vi "Write LinearConfig.vi"(8 "error in (no error)":errorcluster, 10 "LinearConfig":T1={"decoding type"=10092, "units"=10219, "distance per pulse"=0.001, "initial position"=0.0, "z index enable"=FALSE, "z index value"=0.0, "z index phase"=10040} {"units" items=["Meters"=10219, "Inches"=10379, "Ticks"=10304, "From Custom Scale"=10065]; "decoding type" items=["X1"=10090, "X2"=10091, "X4"=10092, "Two Pulse Counting"=10313]; "z index phase" items=["A High B High"=10040, "A High B Low"=10041, "A Low B High"=10042, "A Low B Low"=10043]}, 11 "Linear_Task in":refnum<class "Linear_Task.lvclass">) -> (0 "error out":errorcluster, 3 "Linear_Task out":refnum<class "Linear_Task.lvclass">)   [LabVIEW 2025, in "Linear_Task.lvlib" / "Linear_Task.lvclass"]
uses:
  Linear_Task.lvclass
  Linear_Task.lvclass/Linear_Task.ctl
  DAQ_Module/DAQ_Module/DAQ_Module/DAQ_Linear_Task_Config.ctl
  DAQ_Module/DAQ_Module/DAQ_Module/DAQ_Module.lvclass
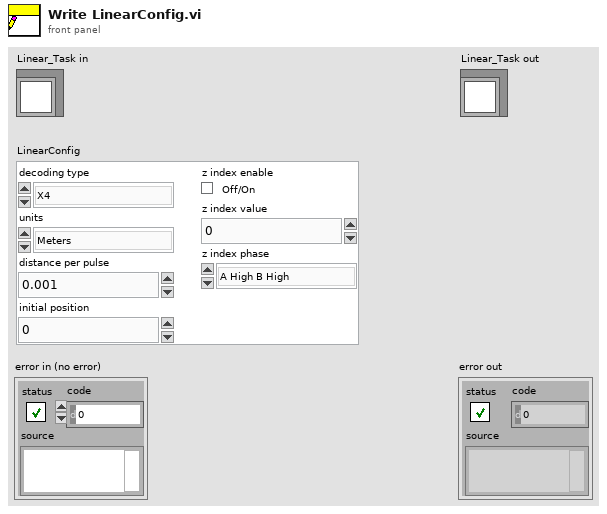
[diagram p1: front panel]
types:
  T1 = typedef "DAQ_Module.lvlib/DAQ_Module.lvclass/DAQ_Linear_Task_Config.ctl" = cluster{"decoding type":i32, "units":i32, "distance per pulse":dbl, "initial position":dbl, "z index enable":bool, "z index value":dbl, "z index phase":i32}
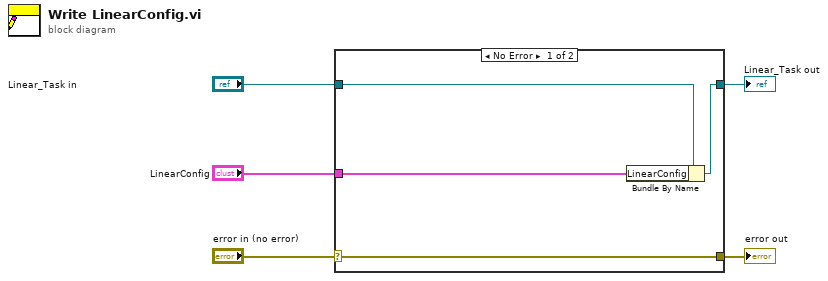
[diagram p0: block diagram]
diagram:
  n1 = case shown="No Error" "error in (no error)" {
    selector: "error in (no error)" -> [w9 w10]
    tunnel: [w9 w10] -> w4
    tunnel: [w7 w11] -> w2
    tunnel: "Linear_Task in" -> [w8 w11]
    tunnel: "LinearConfig" -> [w6 _]
    frame No Error {
      n2 = Bundle By Name(cluster=w8, "LinearConfig"=w6) -> (w7:refnum<class "Linear_Task.lvclass">)
    }
    frame Error {
    }
  }
  "error out" <- w4
  "Linear_Task out" <- w2
